vi "test Set ObjectType_2.vi"(11 "Test Case In":refnum<class "test Electronic Datasheet.lvclass">) -> (0 "error out":errorcluster, 3 "Test Case Out":refnum<class "test Electronic Datasheet.lvclass">)   [LabVIEW 2024, in "test Electronic Datasheet.lvclass"]
uses:
  test Electronic Datasheet.lvclass
  C:/Program Files/National Instruments/LabVIEW 2025/vi.lib/Astemes/LUnit/Test Case.lvclass
  Core/Object Type/Object Type Base.lvclass
  <vilib>/Astemes/LUnit/Test Case.lvclass/Test Case.ctl
  <vilib>/Astemes/LUnit/Append Fail Result.vi
  <vilib>/Astemes/LUnit/Append Pass Result.vi
  <vilib>/Astemes/LUnit/Run In UI.vi
  Core/Value/Value.lvclass
  <vilib>/Astemes/LUnit/Test Case.lvclass
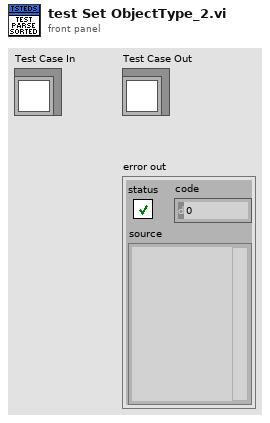
[diagram p1: front panel]
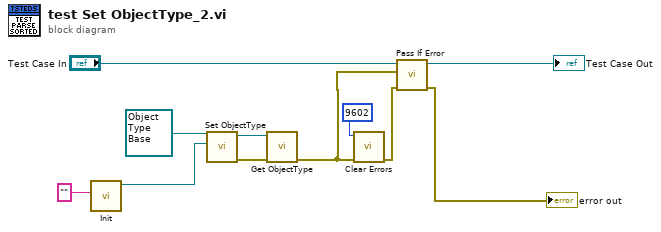
[diagram p0: block diagram]
diagram:
  n1 = call "Init.vi"("Value"="") -> ("Value out"=w7:refnum<class "Value.lvclass">)  [unwired: 9 in, 1 out]
  n2 = call-dynamic "Set ObjectType.vi"("ObjectType"=w7, "Object Type in"=refnum<class "Object Type Base.lvclass"> refnum ("EDS.lvlib:Object Type.lvclass")) -> ("error out"=w5:errorcluster, "Object Type out"=w4:refnum<class "Object Type Base.lvclass">)  [unwired: 8 in]
  n3 = call-dynamic "Get ObjectType.vi"("error in"=w5, "Object Type in"=w4) -> ("error out"=w3:errorcluster)  [unwired: 6 in, 3 out]
  n4 = call <vilib>:"Clear Errors.vi"("error in (no error)"=w3, "specific error code to clear (0: all)"=9602) -> ("error out"=w1:errorcluster)  [unwired: 4 in, 1 out]
  n5 = call <vilib>:"Pass If Error.vi"("error in (no error)"=w1, "Assert error"=w3, "LUnit Test Case In"="Test Case In") -> ("error out"=→"error out":errorcluster, "LUnit Test Case Out"=→"Test Case Out":refnum<class "test Electronic Datasheet.lvclass">)  [unwired: 7 in]
